vi "+cyc2.vi"(1 "% of Cyclic Prefix":dbl format="%#_13g", 2 "Original Signal":cdb[](array[numeric])) -> (0 "Prefixed Signal":cdb[](array[numeric]))   [LabVIEW 2013]
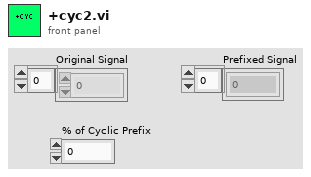
[diagram p1: front panel]
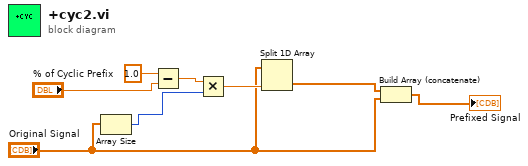
[diagram p0: block diagram]
diagram:
  n1 = Array Size(array="Original Signal") -> (size(s)=w6:i32)
  n2 = Subtract(x=1.0, y="% of Cyclic Prefix") -> (x-y=w5:dbl)
  n3 = Multiply(x=w5, y=w6) -> (x*y=w4:dbl)
  n4 = Split 1D Array(array="Original Signal", index=w4) -> (second subarray=w2:cdb[])  [unwired: 1 out]
  n5 = Build Array (concatenate)(w2, "Original Signal") -> (→"Prefixed Signal":cdb[])
